vi "tuneRightOpenLoop_ShootDualalonSRX.vi"(11 "F Open Loop L":dbl=0.92 format="%.5f") -> ()   [LabVIEW 2019, in "ShootDualTalonSRX_Motor_Pair.lvlib"]
uses:
  ShootDualTalonSRX_Motor_Pair.lvlib
  globals_ShootDualTalonSRX.vi
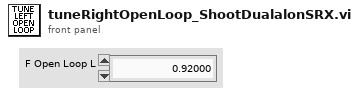
[diagram p1: front panel]
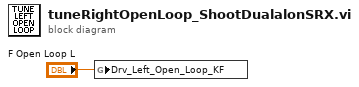
[diagram p0: block diagram]
diagram:
  n1 = global write "globals_ShootDualTalonSRX.vi" "Drv_Left_Open_Loop_KF"("F Open Loop L") -> ()
